vi "Move Fwd PID.vi"(0 "Distance":dbl, 1 "Range":cluster{"output high":dbl, "output low":dbl}={"output high"=1.0, "output low"=0.0} {"output low" format="%.2f"; "output high" format="%.2f"}, 3 "Gains":T1={"proportional gain (Kc)"=1.0, "integral time (Ti, min)"=0.01, "derivative time (Td, min)"=0.0} {"derivative time (Td, min)" format="%.3f"; "integral time (Ti, min)" format="%.3f"; "proportional gain (Kc)" format="%.3f"}, 5 "Encoder Count":dbl, 7 "Reset Rate":bool, 9 "Time to stop":i32=300, 11 "Precision":dbl=0.5 format="%#_13g", 12 "Soft start":dbl=1.0, 14 "Loop Timer":i32=20) -> (4 "Finished?":bool, 15 "Output":dbl)   [LabVIEW 2017]
panel:
  in  "Integral Range":dbl=10000.0
  out "Waveform Chart":cluster{"Distance":dbl, "Encoder Count":dbl}(graph)
  out "rate on?":bool
  # "Time to stop - Tempo que o encoder deve retornar um valor dentro do range da precision para a função considerar que o sistema está parado.\n\nDistance - Setpoint em unidades do encoder.\n\nLoop Timer - Tempo de iteração do loop em que a função está.\n\nPrecision - Range que a função considera \"close enough\" ao setpoint.\n\nEncoder Count - Valor atual do encoder.\n\nRate limit - Limite de aceleração/desaceleração do sistema.\n\nGains - Ganhos do PID.\n\nRange - limite superior e inferior do PID.\n\nSoft Start - constante que aumenta ou diminui o tempo de aceleração no início do movimento"
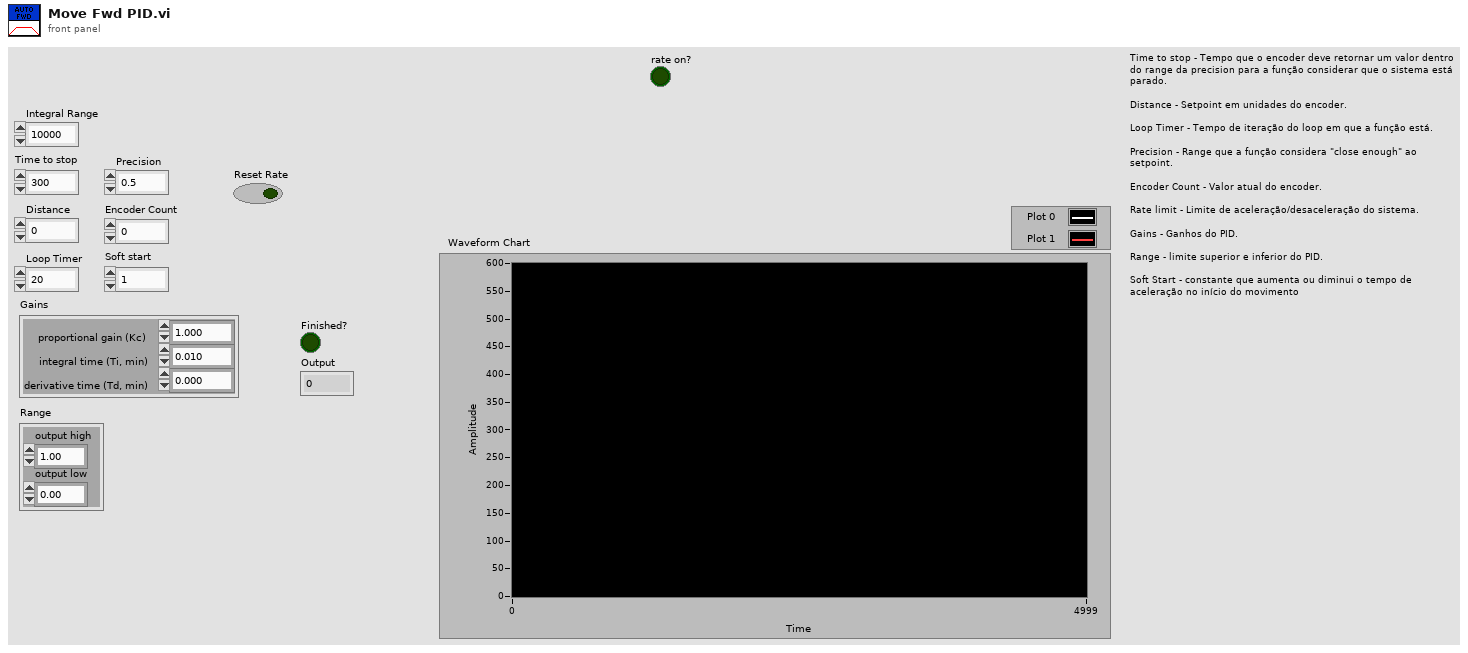
[diagram p1: front panel]
types:
  T1 = cluster{"proportional gain (Kc)":dbl, "integral time (Ti, min)":dbl, "derivative time (Td, min)":dbl}
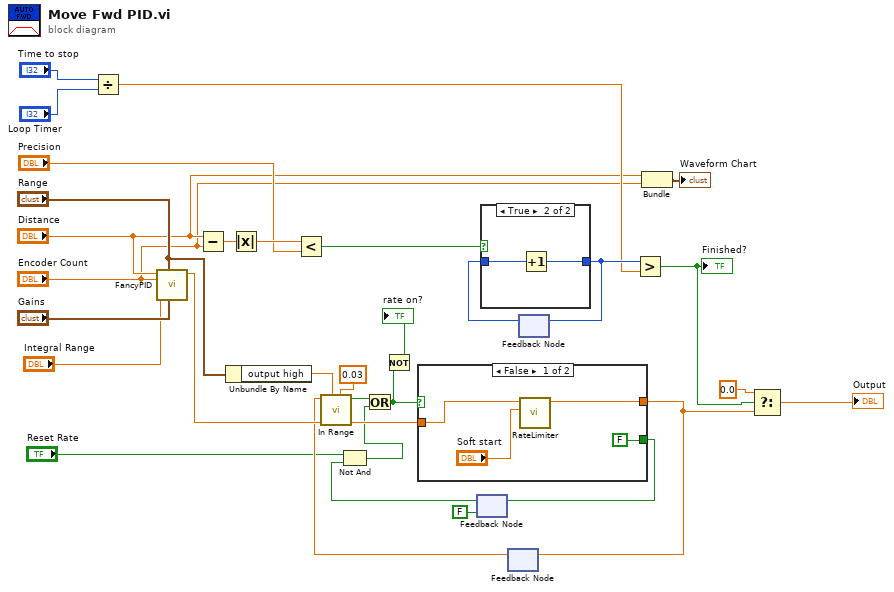
[diagram p0: block diagram]
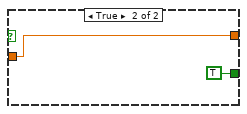
[diagram p2: hidden frame]
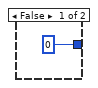
[diagram p3: hidden frame]
diagram:
  n1 = Divide(x="Time to stop", y="Loop Timer") -> (x/y=w25:dbl)
  n2 = call "FancyPID.vi"("Gains"="Gains", "Range"="Range", "Integral Range"="Integral Range", "Process variable"="Encoder Count", "Setpoint"="Distance") -> ("output"=w14:dbl)  [unwired: 6 in]
  n3 = Subtract(x="Distance", y="Encoder Count") -> (x-y=w24:dbl)
  n4 = Unbundle By Name("Range") -> ("output high"=w20:dbl)
  n5 = Absolute Value(x=w24) -> (abs(x)=w30:dbl)
  n6 = Less?(x=w30, y="Precision") -> (x < y?=w28:bool)
  n7 = feedback #1(FALSE) -> (w8:bool)
  n8 = Not And(1:w8, 2:"Reset Rate") -> (0:w7:bool)
  n9 = feedback #2() -> (w13:dbl)  [unwired: 1 in]
  n10 = call "In Range.vi"("Range"=0.03, "Setpoint"=w20, "Value"=w13) -> ("in range?"=w18:bool)  [unwired: 8 in]
  n11 = Or(x=w18, y=w7) -> (x .or. y?=w17:bool)
  n12 = Not(x=w17) -> (.not. x?=→"rate on?":bool)
  n13 = case shown="False" w17 {
    tunnel: [w35 w36] -> w12
    tunnel: w14 -> [w34 w36]
    tunnel: [FALSE TRUE] -> w16
    frame False {
      n14 = call "RateLimiter.vi"("Max dx/dt"="Soft start", "Input"=w34) -> ("Output"=w35:dbl)  [unwired: 9 in]
    }
    frame True {
    }
  }
  n15 = feedback-in #1(w16) -> ()
  n16 = feedback-in #2(w12) -> ()
  n17 = feedback #3() -> (w27:i32)  [unwired: 1 in]
  n18 = case shown="True" w28 {
    tunnel: [0 w40] -> w26
    tunnel: w27 -> [_ w39]
    frame False {
    }
    frame True {
      n19 = Increment(x=w39) -> (x+1=w40:i32)
    }
  }
  n20 = feedback-in #3(w26) -> ()
  n21 = Greater?(x=w26, y=w25) -> (0:w9:bool)
  "Finished?" <- w9
  n22 = Bundle("Distance"="Distance", "Encoder Count"="Encoder Count") -> (→"Waveform Chart":cluster{"Distance":dbl, "Encoder Count":dbl})  [unwired: 1 in]
  n23 = Select(t=0.0, s=w9, f=w12) -> (s? t:f=→"Output":dbl)
